vi "setGainByToken.vi"(6 "Delay between send and receive [ms]":i32=100, 8 "error in (no error)":errorcluster, 11 "CCD in":refnum<class "CCD.lvclass">) -> (0 "error out":errorcluster, 1 "ID":i32, 2 "results-JSON string":string, 3 "CCD out":refnum<class "CCD.lvclass">)   [LabVIEW 2023]
uses:
  CCD.lvclass
  20f7d3bd-08ac-4524-9bed-df36c1da25a0.vi
  5b02aa1a-f403-4d30-91c8-1c594f70e61d.vi
  <vilib>/JDP Science/JSONtext/Variant to JSON Text.vi
  <vilib>/JDP Science/JSONtext/Set Item.vi
  <vilib>/JDP Science/JSONtext/LVClass Serializer/JSONtext LVClass Serializer.lvclass
  GenericDevice/GenericDevice.lvclass
  <vilib>/IlluminatedG/lv-web-crypto/lv-json/JSON/JSON.lvlib
panel:
  in  "gain token":u16
  # "Connector Pane"
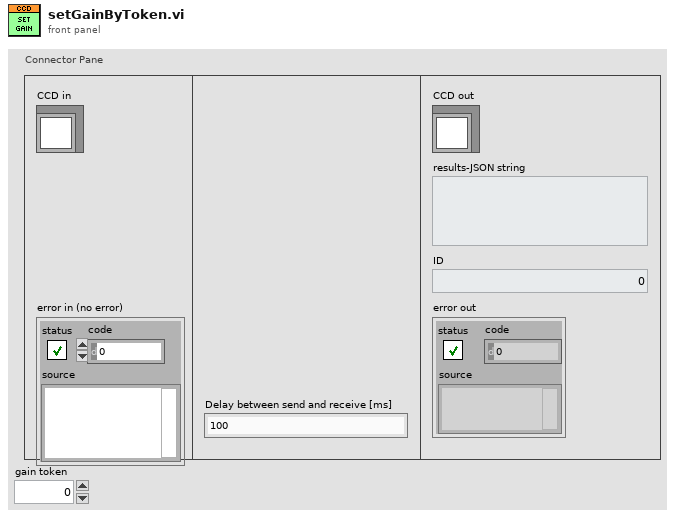
[diagram p1: front panel]
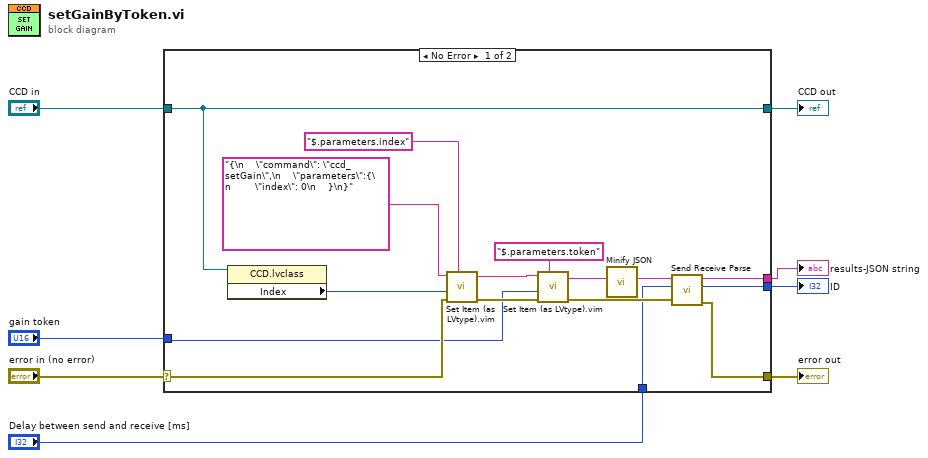
[diagram p0: block diagram]
diagram:
  n1 = case shown="No Error" "error in (no error)" {
    selector: "error in (no error)" -> [w21 w26]
    tunnel: [w17 w26] -> w7
    tunnel: [w11 w25] -> w5
    tunnel: "CCD in" -> [w11 w25]
    tunnel: "gain token" -> [w9 _]
    tunnel: [w15 _] -> w4
    tunnel: [w16 _] -> w3
    tunnel: "Delay between send and receive [ms]" -> [w10 _]
    frame No Error {
      n2 = property class="CCD.lvclass"(reference=w11) -> ("Index"=w22:i32)  [unwired: 1 in, 2 out]
      n3 = call "Set Item (as LVtype).vim"("$Path or Item Name"="$.parameters.index", "error in (no error)"=w21, "Anything"=w22, "JSON"="{\n    \"command\": \"ccd_setGain\",\n    \"parameters\":{\n        \"index\": 0\n    }\n}") -> ("error out"=w12:errorcluster, "<JSON>"=w20:string)  [unwired: 4 in, 1 out]
      n4 = call "Set Item (as LVtype).vim"("$Path or Item Name"="$.parameters.token", "error in (no error)"=w12, "Anything"=w9, "JSON"=w20) -> ("error out"=w19:errorcluster, "<JSON>"=w14:string)  [unwired: 4 in, 1 out]
      n5 = call <vilib>:"Minify JSON.vi"("JSON String"=w14) -> ("Minified JSON"=w13:string)  [unwired: 10 in]
      n6 = call "Send Receive Parse.vi"("error in"=w19, "Delay between send and receive [ms]"=w10, "<JSON>"=w13) -> ("error out"=w17:errorcluster, "ID"=w16:i32, "results-JSON string"=w15:string)  [unwired: 6 in]
    }
    frame Error {
    }
  }
  "error out" <- w7
  "CCD out" <- w5
  "results-JSON string" <- w4
  "ID" <- w3
